vi "Test.vi"() -> ()   [LabVIEW 2017]
doc: "This VI is called when test mode begins, and will automatically be terminated when it ends. You can add manual or automatic tests and invoke them from the dashboard."
uses:
  Intake/Intake Notifier.ctl
  Intake/Intake Control Type.ctl
  Lift/Lift Notifier.ctl
  Lift/Lift Control Type.ctl
  Lift/Lift Enum States.ctl
  Drive/Drive Notifier.ctl
  Drive/Drive Control Type.ctl
  RPED/RPED Notifier.ctl
  RPED/RPED Control Type.ctl
  Intake Rotation/Intake Rotation Notifier.ctl
  Intake Rotation/Intake Rotation Control Type.ctl
  Intake Rotation/Arm Enum States.ctl
  Drive/Drive Globals.vi
  Lift/Lift Globals.vi
  Intake/Intake Globals.vi
  RPED/RPED Globals.vi
  Intake Rotation/Intake Rotation Globals.vi
  Utility VIs/Refnum Names.vi
  <vilib>/Rock Robotics/WPI/Utilities/WPI_GetSetVariantRefNum.vi
panel:
  out "error out 5":errorcluster
  out "error out 4":errorcluster
  out "error out 3":errorcluster
  out "error out 2":errorcluster
  out "error out":errorcluster
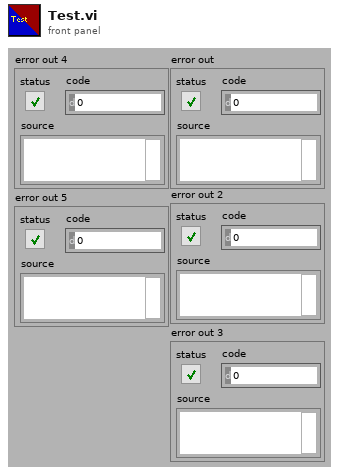
[diagram p1: front panel]
types:
  T1 = typedef "Intake Rotation Notifier.ctl" = cluster{"Step":i32, "Intake Rotation Control Type":T2, "Parameter 1":dbl, "Parameter 2":dbl, "Intake Rotation Notifier":refnum<notifier>, "Manual Up":bool, "Manual Down":bool, "Climb":bool, "Switch":bool, "Scale Low":bool, "Scale High":bool, "Stow":bool, "Load":bool, "Scale Mid":bool, "Exchange":bool, "Set Position":T3, "Portal":bool}
  T2 = typedef "Intake Rotation Control Type.ctl" = enum16{"No Op", "Manual Up", "Position", "Manual Down", "PositionAuto"}
  T3 = typedef "Arm Enum States.ctl" = enum16{"Current Position", "Climb", "Load", "Portal", "Switch", "Scale High", "Scale Mid", "Scale Low", "Exchange", "Stow"}
  T4 = typedef "RPED Notifier.ctl" = cluster{"RPED Control Type":T5, "Step":i32, "Left Forward":bool, "Right Forward":bool, "Parameter 1":dbl, "Parameter 2":dbl, "Parameter 3":dbl, "RPED Notifier":refnum<notifier>, "Left Back":bool, "Right Back":bool, "Right":bool, "Left":bool}
  T5 = typedef "RPED Control Type.ctl" = enum16{"No Op", "Left Manual", "Right Manual", "Time", "Left", "Right", "Left_Slow", "Right_Slow", "Left_Distance", "Right_Distance"}
  T6 = typedef "Drive Notifier.ctl" = cluster{"Drive Control Type":T7, "Throttle":dbl, "Twist":dbl, "Step":i32, "High Gear":bool, "Parameter 1":dbl, "Parameter 2":dbl, "Parameter 3":dbl, "Drive Notifier":refnum<notifier>, "AutoTrack":bool}
  T7 = typedef "Drive Control Type.ctl" = enum16{"No_Op", "Basic Drive", "Time", "Heading", "Hybrid_Turn", "RC_Speed", "Switch_Slots", "AutoTrack_Cube", "Speed Test", "Turn_Cube", "To_Cube", "Wait", "Distance_Slow", "Distance", "D_H_Delay", "Distance_Delay", "Heading_Cap", "Heading_Tight", "Cube_Heading", "Distance_Ramp"}
  T8 = typedef "Lift Notifier.ctl" = cluster{"Lift Control Type":T9, "Step":i32, "Set Position":T10, "Climb":bool, "Switch":bool, "Scale Low":bool, "Scale Mid":bool, "Scale High":bool, "Stow":bool, "Load":bool, "Climb Actuation":bool, "Manual Up":bool, "Manual Down":bool, "Parameter 1":dbl, "Parameter 2":dbl, "Parameter 3":dbl, "Lift Notifier":refnum<notifier>, "Exchange":bool, "Brake":bool, "Portal":bool}
  T9 = typedef "Lift Control Type.ctl" = enum16{"No Op", "Position", "Climb Actuation", "Manual Up", "Manual Down", "PositionAuto", "Position_kP", "Position_Delay"}
  T10 = typedef "Lift Enum States.ctl" = enum16{"Climb", "Load", "Portal", "Switch", "Scale High", "Scale Mid", "Scale Low", "Exchange", "Stow", "Current Position"}
  T11 = typedef "Intake Notifier.ctl" = cluster{"Intake Control Type":T12, "Step":i32, "In":bool, "Speed":dbl, "Out":bool, "Parameter 1":dbl, "Parameter 2":dbl, "Intake Notifier":refnum<notifier>, "Actuate Cube":bool, "Speed In":dbl, "Speed Out":dbl, "Load":bool, "Override":bool, "Exchange":bool, "Intake Open":bool}
  T12 = typedef "Intake Control Type.ctl" = enum16{"No Op", "In", "Out", "Test Mode", "Cube_In", "Cube_Out", "State_Change"}
  T13 = typedef "Joystick Controls.ctl" = cluster{"Pilot Left Joystick X":dbl, "Pilot Left Joystick Y":dbl, "Pilot A Button":bool, "Pilot B Button":bool, "Pilot X Button":bool, "Pilot Y Button":bool, "Pilot Left Bumper":bool, "Pilot Right Bumper":bool, "Pilot View Button":bool, "Pilot Menu Button":bool, "Pilot Left Joystick Press":bool, "Pilot Right Joystick Press":bool, "Pilot Left Trigger":dbl, "Pilot Right Joystick X":dbl, "Pilot Right Joystick Y":dbl, "Pilot Right Trigger":dbl, "Copilot Left Joystick X":dbl, "Copilot Left Joystick Y":dbl, "Copilot A Button":bool, "Copilot B Button":bool, "Copilot X Button":bool, "Copilot Y Button":bool, "Copilot Left Bumper":bool, "Copilot Right Bumper":bool, "Copilot View Button":bool, "Copilot Menu Button":bool, "Copilot Left Joystick Press":bool, "Copilot Right Joystick Press":bool, "Copilot Left Trigger":dbl, "Copilot Right Joystick X":dbl, "Copilot Right Joystick Y":dbl, "Copilot Right Trigger":dbl, "Pilot D-Pad":i16, "Copilot D-Pad":i16}
  T14 = typedef "WPI_CompressorDevRef.ctl" = cluster{"DevStatus":errorcluster, "Pneumatics Control Module":u8}
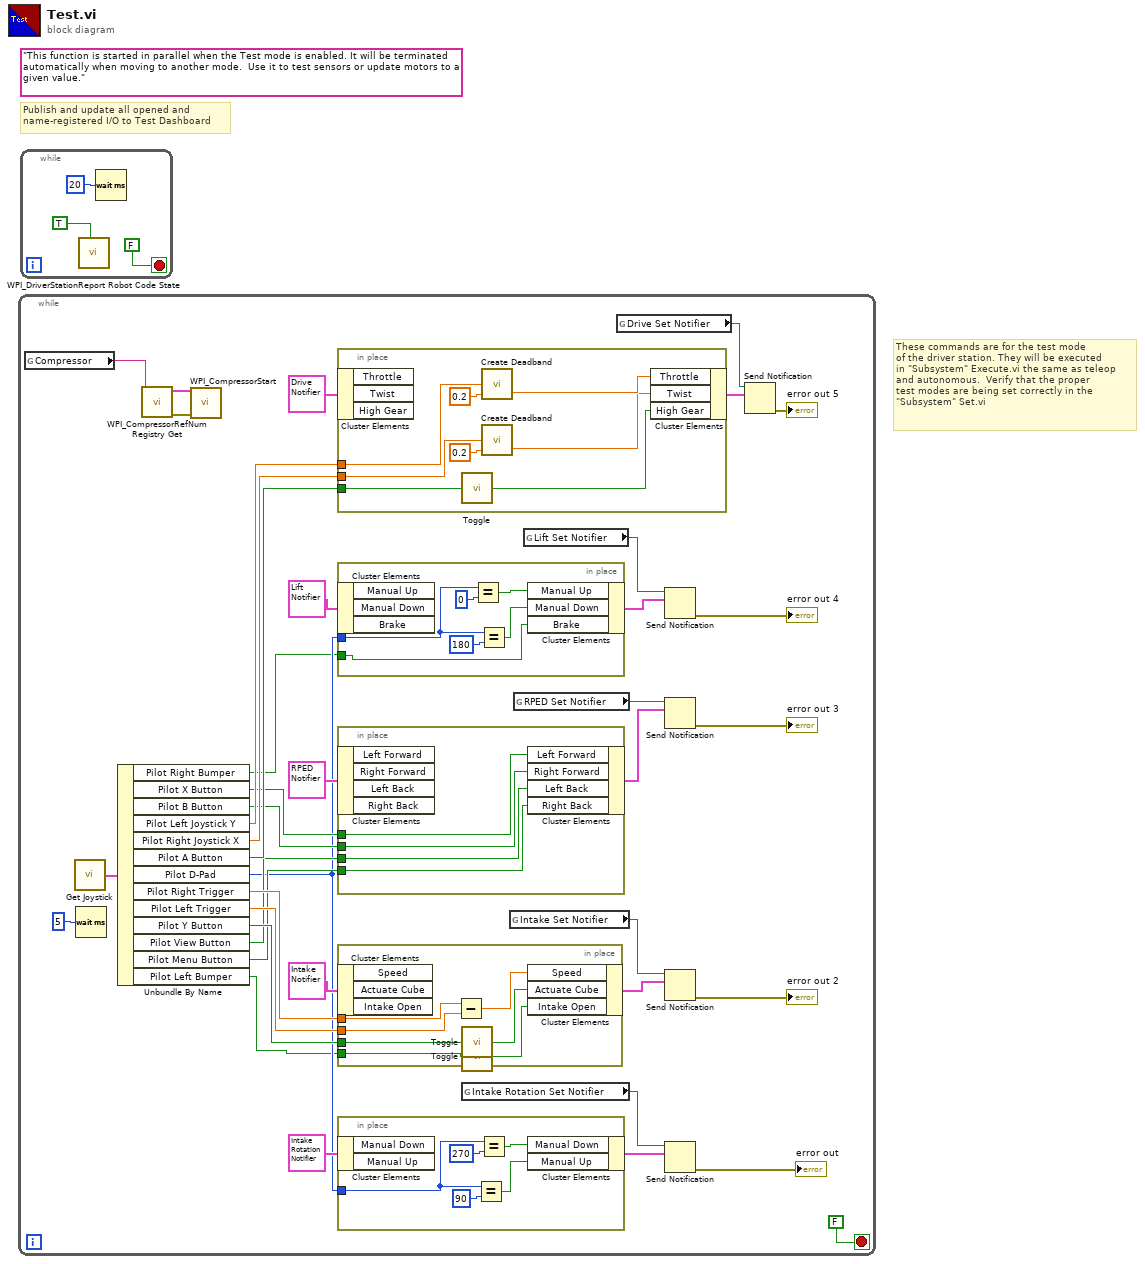
[diagram p0: block diagram]
diagram:
  (unwired) "This function is started in parallel when the Test mode is enabled. It will be terminated automatically when moving to another mode.  Use it to test sensors or update motors to a given value."
  # "These commands are for the test mode\nof the driver station. They will be executed\nin \"Subsystem\" Execute.vi the same as teleop \nand autonomous.  Verify that the proper\ntest modes are being set correctly in the \n\"Subsystem\" Set.vi"
  # "Publish and update all opened and\nname-registered I/O to Test Dashboard"
  n1 = while {
    stop <- FALSE stop-if-true
    n2 = global read "Refnum Names.vi" "Compressor"() -> (w4:string)
    n3 = call "Get Joystick.vi"() -> ("Joystick Controls"=w39:T13)  [unwired: 7 in]
    n4 = Wait (ms)(milliseconds to wait=u32 5) -> ()  [unwired: 1 out]
    n5 = Unbundle By Name(w39) -> ("Pilot Right Bumper"=w5:bool, "Pilot X Button"=w23:bool, "Pilot B Button"=w22:bool, "Pilot Left Joystick Y"=w27:dbl, "Pilot Right Joystick X"=w26:dbl, "Pilot A Button"=w25:bool, "Pilot D-Pad"=w6:i16, "Pilot Right Trigger"=w21:dbl, "Pilot Left Trigger"=w20:dbl, "Pilot Y Button"=w17:bool, "Pilot View Button"=w13:bool, "Pilot Menu Button"=w12:bool, "Pilot Left Bumper"=w1:bool)
    n6 = call <vilib>:"WPI_CompressorRefNum Registry Get.vi"("refnum name"=w4) -> ("error out"=w2:errorcluster, "CompressorDevRef"=w3:T14)  [unwired: 9 in]
    n7 = call <vilib>:"WPI_CompressorStart.vi"("error in (no error)"=w2, "CompressorDevRef"=w3) -> ()  [unwired: 8 in, 2 out]
    n8 = in-place {
      in-place-border: w27 -> [w65]
      in-place-border: w26 -> [w64]
      in-place-border: w25 -> [w68]
      n9 = in-place-cluster #1(T6 {"Drive Control Type"=enum."No_Op", "Throttle"=0.0, "Twist"=0.0, "Step"=0, "High Gear"=FALSE, "Parameter 1"=0.0, "Parameter 2"=0.0, "Parameter 3"=0.0, "Drive Notifier"=refnum, "AutoTrack"=FALSE} ("Drive Notifier")) -> ()  [unwired: 3 out]
      n10 = call "Toggle.vi"("Boolean"=w68) -> ("Boolean Out"=w69:bool)
      n11 = call "Create Deadband.vi"("Input Deadband"=0.2, "Input"=w65) -> ("Output"=w67:dbl)  [unwired: 2 in]
      n12 = call "Create Deadband.vi"("Input Deadband"=0.2, "Input"=w64) -> ("Output"=w66:dbl)  [unwired: 2 in]
      n13 = in-place-cluster #1("Throttle"=w67, "Twist"=w66, "High Gear"=w69) -> (w38:T6)
    }
    n14 = in-place {
      in-place-border: w6 -> [w50]
      in-place-border: w5 -> [w49]
      n15 = in-place-cluster #2(T8 {"Lift Control Type"=enum."No Op", "Step"=0, "Set Position"=enum."Load", "Climb"=FALSE, "Switch"=FALSE, "Scale Low"=FALSE, "Scale Mid"=FALSE, "Scale High"=FALSE, "Stow"=FALSE, "Load"=FALSE, "Climb Actuation"=FALSE, "Manual Up"=FALSE, "Manual Down"=FALSE, "Parameter 1"=0.0, "Parameter 2"=0.0, "Parameter 3"=0.0, "Lift Notifier"=refnum, "Exchange"=FALSE, "Brake"=FALSE, "Portal"=FALSE} ("Lift Notifier")) -> ()  [unwired: 3 out]
      n16 = Equal?(x=w50, y=i16 0) -> (x = y?=w54:bool)
      n17 = Equal?(x=w50, y=i16 180) -> (x = y?=w53:bool)
      n18 = in-place-cluster #2("Manual Up"=w54, "Manual Down"=w53, "Brake"=w49) -> (w36:T8)
    }
    n19 = in-place {
      in-place-border: w23 -> [w48]
      in-place-border: w22 -> [w47]
      in-place-border: w13 -> [w46]
      in-place-border: w12 -> [w45]
      n20 = in-place-cluster #3(T4 {"RPED Control Type"=enum."No Op", "Step"=0, "Left Forward"=FALSE, "Right Forward"=FALSE, "Parameter 1"=0.0, "Parameter 2"=0.0, "Parameter 3"=0.0, "RPED Notifier"=refnum, "Left Back"=FALSE, "Right Back"=FALSE, "Right"=FALSE, "Left"=FALSE} ("RPED Notifier")) -> ()  [unwired: 4 out]
      n21 = in-place-cluster #3("Left Forward"=w48, "Right Forward"=w47, "Left Back"=w46, "Right Back"=w45) -> (w30:T4)
    }
    n22 = in-place {
      in-place-border: w21 -> [w59]
      in-place-border: w20 -> [w60]
      in-place-border: w17 -> [w57]
      in-place-border: w1 -> [w55]
      n23 = in-place-cluster #4(T11 {"Intake Control Type"=enum."No Op", "Step"=0, "In"=FALSE, "Speed"=0.0, "Out"=FALSE, "Parameter 1"=0.0, "Parameter 2"=0.0, "Intake Notifier"=refnum, "Actuate Cube"=FALSE, "Speed In"=0.0, "Speed Out"=0.0, "Load"=FALSE, "Override"=FALSE, "Exchange"=FALSE, "Intake Open"=FALSE} ("Intake Notifier")) -> ()  [unwired: 3 out]
      n24 = Subtract(x=w59, y=w60) -> (x-y=w61:dbl)
      n25 = call "Toggle.vi"("Boolean"=w57) -> ("Boolean Out"=w58:bool)
      n26 = call "Toggle.vi"("Boolean"=w55) -> ("Boolean Out"=w56:bool)
      n27 = in-place-cluster #4("Speed"=w61, "Actuate Cube"=w58, "Intake Open"=w56) -> (w37:T11)
    }
    n28 = in-place {
      in-place-border: w6 -> [w40]
      n29 = in-place-cluster #5(T1 {"Step"=0, "Intake Rotation Control Type"=enum."No Op", "Parameter 1"=0.0, "Parameter 2"=0.0, "Intake Rotation Notifier"=refnum, "Manual Up"=FALSE, "Manual Down"=FALSE, "Climb"=FALSE, "Switch"=FALSE, "Scale Low"=FALSE, "Scale High"=FALSE, "Stow"=FALSE, "Load"=FALSE, "Scale Mid"=FALSE, "Exchange"=FALSE, "Set Position"=enum."Climb", "Portal"=FALSE} ("Intake Rotation Notifier")) -> ()  [unwired: 2 out]
      n30 = Equal?(x=w40, y=i16 90) -> (x = y?=w41:bool)
      n31 = Equal?(x=w40, y=i16 270) -> (x = y?=w43:bool)
      n32 = in-place-cluster #5("Manual Down"=w43, "Manual Up"=w41) -> (w15:T1)
    }
    n33 = global read "Intake Rotation Globals.vi" "Intake Rotation Set Notifier"() -> (w14:refnum<notifier>)
    n34 = global read "Intake Globals.vi" "Intake Set Notifier"() -> (w31:refnum<notifier>)
    n35 = global read "RPED Globals.vi" "RPED Set Notifier"() -> (w28:refnum<notifier>)
    n36 = global read "Lift Globals.vi" "Lift Set Notifier"() -> (w32:refnum<notifier>)
    n37 = global read "Drive Globals.vi" "Drive Set Notifier"() -> (w34:refnum<notifier>)
    n38 = Send Notification(notification=w36, notifier=w32) -> (error out=→"error out 4":errorcluster)  [unwired: 1 in, 1 out]
    n39 = Send Notification(notification=w30, notifier=w28) -> (error out=→"error out 3":errorcluster)  [unwired: 1 in, 1 out]
    n40 = Send Notification(notification=w37, notifier=w31) -> (error out=→"error out 2":errorcluster)  [unwired: 1 in, 1 out]
    n41 = Send Notification(notification=w15, notifier=w14) -> (error out=→"error out":errorcluster)  [unwired: 1 in, 1 out]
    n42 = Send Notification(notification=w38, notifier=w34) -> (error out=→"error out 5":errorcluster)  [unwired: 1 in, 1 out]
  }
  n43 = while {
    stop <- FALSE stop-if-true
    n44 = call <vilib>:"WPI_DriverStationReport Robot Code State.vi"("Test"=TRUE ("Autonomous")) -> ()  [unwired: 10 in, 1 out]
    n45 = Wait (ms)(milliseconds to wait=u32 20) -> ()  [unwired: 1 out]
  }
